vi "Get voltage.vi"(8 "Measurement data in":T1, 11 "Byte array":u8[](array[numeric])) -> (0 "Measurement data out":T1, 3 "Byte array":u8[](array[numeric]))   [LabVIEW 2020]
uses:
  Typedefs/Measurement data.ctl
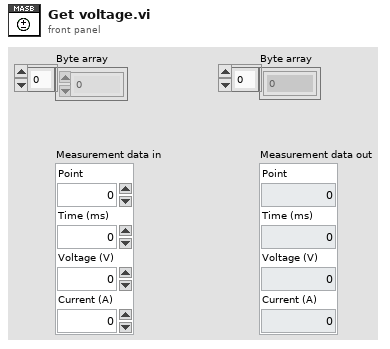
[diagram p1: front panel]
types:
  T1 = typedef "Measurement data.ctl" = cluster{"Point":u32, "Time (ms)":u32, "Voltage (V)":dbl, "Current (A)":dbl}
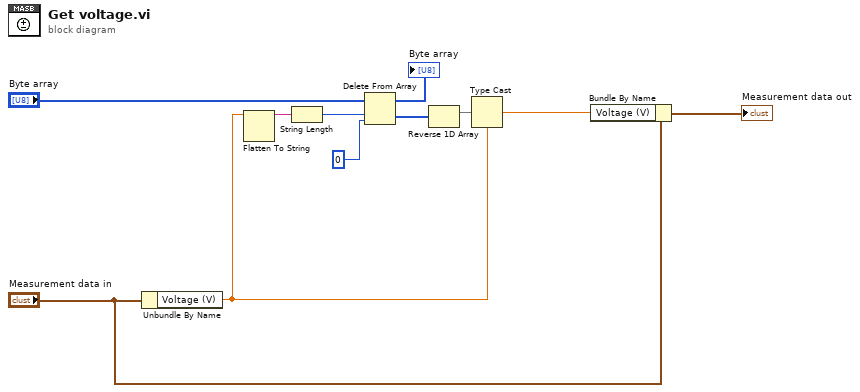
[diagram p0: block diagram]
diagram:
  n1 = Unbundle By Name("Measurement data in") -> ("Voltage (V)"=w8:dbl)
  n2 = Flatten To String(anything=w8) -> (data string=w5:string)  [unwired: 3 in, 2 out]
  n3 = String Length(string=w5) -> (length=w6:i32)
  n4 = Delete From Array(array="Byte array", length=w6, index=0) -> (deleted portion=w7:u8[], array with subset deleted=→"Byte array":u8[])
  n5 = Reverse 1D Array(array=w7) -> (reversed array=w2:u8[])
  n6 = Type Cast(type=w8, x=w2) -> (*(type *) &x=w10:dbl)
  n7 = Bundle By Name(cluster="Measurement data in", "Voltage (V)"=w10) -> (→"Measurement data out":T1)
